vi "Get Clicked Array Index.vi"() -> ()   [LabVIEW 2017]
doc: "This example shows how to determine which element of an array a user has clicked on the front panel. It uses an even structure to determine when a user has clicked on an array element. Then using the coordinates of the mouse cursor and the dimensions of the array, it calculates which element was clicked on."
panel:
  out "Clicked Index":i32[](array[numeric])
  in  "stop":bool
  in  "Array":dbl[][](array[numeric])
  # "EXAMPLE DOWNLOADED -- DOESN'T WORK EXACTLY, NEITHER FOR ME!"
  # "Overview: This example shows how to determine which element of an array a user has clicked on the front panel.\n\nRequirements: LabVIEW 2012\n\nInstructions:\n1. Run the VI.\n2. Click on a cell in the array.\n3. Compare the result from the indicator \"Clicked Index\"."
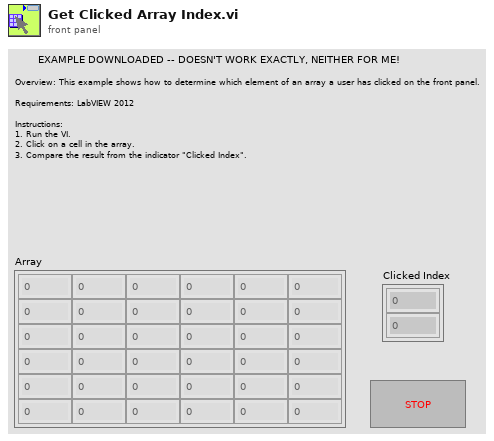
[diagram p1: front panel]
types:
  T1 = typedef "LVPositionTypeDef.ctl" = cluster{"Left":i32, "Top":i32}
  T2 = typedef "LVBoundsTypeDef.ctl" = cluster{"Width":u32, "Height":u32}
  T3 = typedef "LVPoint32TypeDef.ctl" = cluster{"Horizontal":i32, "Vertical":i32}
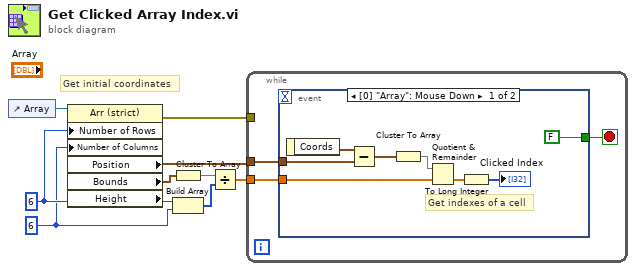
[diagram p0: block diagram]
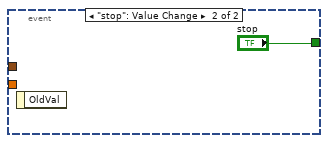
[diagram p2: hidden frame]
diagram:
  w5 = u32 6 ("dimension size")
  w6 = u32 6 ("dimension size")
  # "Get initial coordinates"
  n1 = control-ref of="Array"() -> (w9:refnum<vi>)
  n2 = property on="Property Node" class="Arr (strict)" props=["Number of Rows", "Number of Columns", "Position", "Bounds", "Height"](reference=w9, "Number of Rows"=w6, "Number of Columns"=w5) -> (error out=w8:errorcluster, "Position"=w1:T1, "Bounds"=w7:T2)  [unwired: 1 in, 2 out]
  n3 = Cluster To Array(cluster=w7) -> (array=w4:u32[])
  n4 = Build Array(w6, w5) -> (w3:u32[])
  n5 = Divide(x=w4, y=w3) -> (x/y=w2:dbl[])
  n6 = while {
    tunnel: w8 -> [_]
    tunnel: w2 -> [w12]
    tunnel: w1 -> [w10]
    stop <- w11 stop-if-true
    n7 = event shown="[0] \"Array\": Mouse Down" {
      selector: _ -> [_ _]
      dyn-events: _ -> [_ _]
      timeout: _ -> [_ _]
      tunnel: w12 -> [w16 _]
      tunnel: [FALSE ("stop") "stop"] -> w11
      tunnel: w10 -> [w19 _]
      event "Array": Mouse Down {
        # "Get indexes of a cell"
        n8 = event-data() -> ("Coords"=w18:T3)  [unwired: 1 in]
        n9 = Subtract(x=w18, y=w19) -> (x-y=w14:T3)
        n10 = Cluster To Array(cluster=w14) -> (array=w17:i32[])
        n11 = Quotient & Remainder(x=w17, y=w16) -> (floor(x/y)=w15:dbl[])  [unwired: 1 out]
        n12 = To Long Integer(number=w15) -> (32bit integer=→"Clicked Index":i32[])
      }
      event "stop": Value Change {
        n13 = event-data() -> ()  [unwired: 1 in, 1 out]
      }
    }
  }
